vi "Decorder.vi"(0 "A1":bool) -> (1 "D3":bool, 2 "D2":bool, 3 "D1":bool)   [LabVIEW 2022 SP3]
panel:
  out "D0":bool
  in  "A0":bool
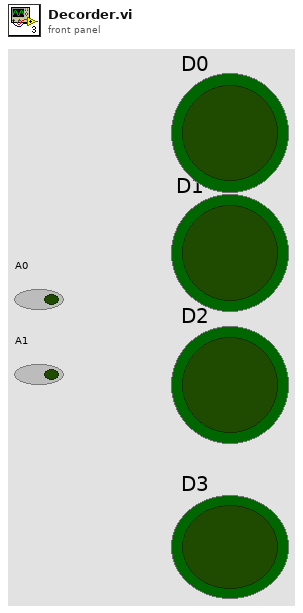
[diagram p1: front panel]
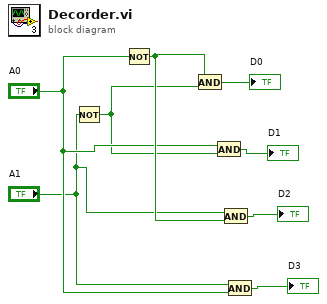
[diagram p0: block diagram]
diagram:
  n1 = Not(x="A1") -> (.not. x?=w5:bool)
  n2 = Not(x="A0") -> (.not. x?=w8:bool)
  n3 = And(x=w8, y=w5) -> (x .and. y?=→"D0":bool)
  n4 = And(x="A0", y=w5) -> (x .and. y?=→"D1":bool)
  n5 = And(x="A1", y=w8) -> (x .and. y?=→"D2":bool)
  n6 = And(x="A1", y="A0") -> (x .and. y?=→"D3":bool)
